vi "Configure Measurement.vi"(8 "error in (no error)":errorcluster, 11 "Mag Lab Measurement in":refnum<class "Mag Lab Measurement.lvclass">) -> (0 "error out":errorcluster, 3 "Mag Lab Measurement out":refnum<class "Mag Lab Measurement.lvclass">)   [LabVIEW 2015, in "Mag Lab Measurement.lvclass"]
uses:
  Mag Lab Measurement.lvclass
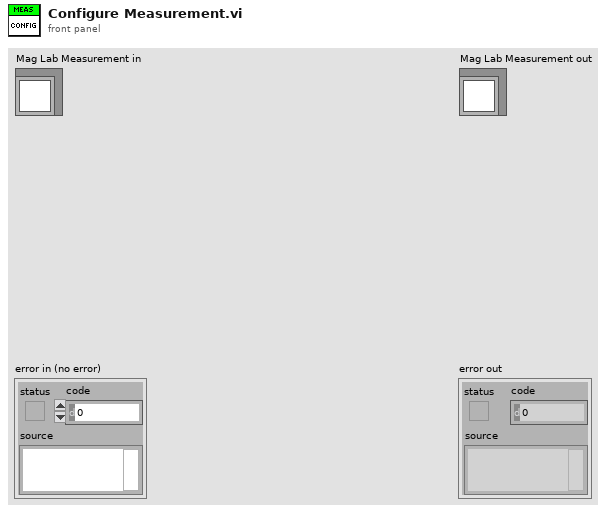
[diagram p1: front panel]
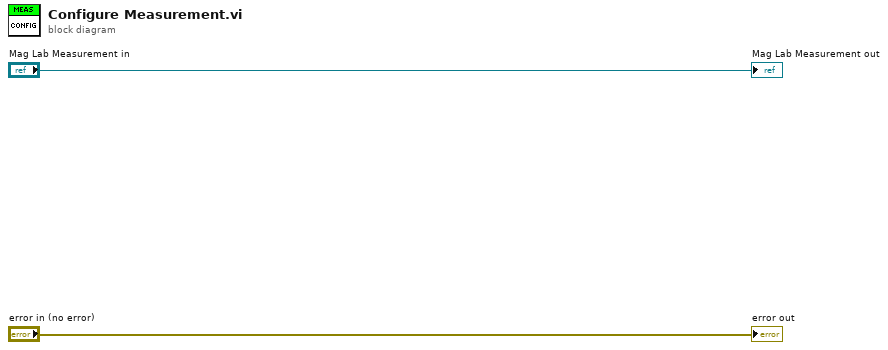
[diagram p0: block diagram]
diagram:
  "error out" <- "error in (no error)"
  "Mag Lab Measurement out" <- "Mag Lab Measurement in"
